vi "Read-Write File Paths setup-Write key.vi"(4 "Type":T1, 5 "Section":string, 6 "Which file or folder?":T3, 7 "Key":string, 8 "error in (no error)":errorcluster, 9 "error in":errorcluster, 10 "Value in":string, 11 "Refnum in":T2) -> (0 "error out":errorcluster, 2 "Value out":string, 3 "Refnum out":T2)   [LabVIEW 2013]
uses:
  Typedefs/Which path.ctl
  <vilib>/Utility/config.llb/Config Data RefNum.ctl
  Typedefs/File or Folder path or name.ctl
  <vilib>/Utility/config.llb/Write Key (String).vi
  <vilib>/Utility/config.llb/NI_LVConfig.lvlib
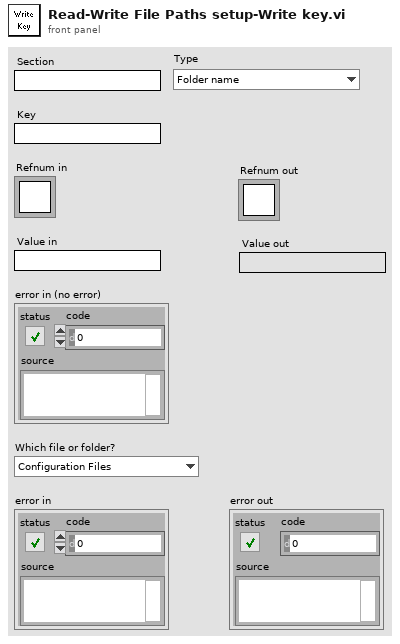
[diagram p1: front panel]
types:
  T1 = typedef "File or Folder path or name.ctl" = enum16{"Folder name", "Folder path", "File name", "File path & name"}
  T2 = typedef "NI_LVConfig.lvlib/Config Data RefNum.ctl" = refnum<k1>
  T3 = typedef "Which path.ctl" = enum16{"Configuration Files", "Calibration Files", "Images", "Setup.ini", "Loaded User profile.ini", "User's-Previous session.ini", "New user profile.ini", "Selected User profile.ini", "User profiles folder", "Power meter scaling.txt", "FOV Cal.ini"}
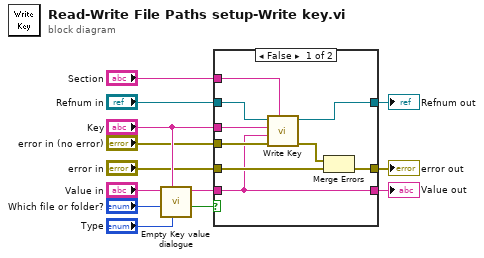
[diagram p0: block diagram]
diagram:
  n1 = call "Empty Key value dialogue.vi"("Type"="Type", "Key"="Key", "Which file or folder?"="Which file or folder?", "Key's value in"="Value in") -> ("Cancel"=w12:bool, "Key's value out"=w10:string)  [unwired: 6 in]
  n2 = case shown="False" w12 {
    tunnel: "Section" -> [w22 _]
    tunnel: "Refnum in" -> [w21 w25]
    tunnel: "error in (no error)" -> [w20 _]
    tunnel: [w19 w25] -> w6
    tunnel: [w17 w24] -> w7
    tunnel: "error in" -> [w16 w24]
    tunnel: w10 -> [w14 w23]
    tunnel: "Key" -> [w15 _]
    tunnel: [w14 w23] -> w2
    frame False {
      n3 = call-poly <vilib>:"Write Key.vi"("section"=w22, "error in (no error)"=w20, "value"=w14, "key"=w15, "refnum"=w21) -> ("error out"=w18:errorcluster, "refnum out"=w19:T2)  [unwired: 4 in, 1 out]
      n4 = Merge Errors(w18, w16) -> (w17:errorcluster)
    }
    frame True {
    }
  }
  "error out" <- w7
  "Refnum out" <- w6
  "Value out" <- w2
